vi "QueryTarget.vi"(8 "error in (no error)":errorcluster, 11 "Target Reference in":refnum<k24>) -> (0 "error out":errorcluster, 2 "Target Information":T1, 3 "Target Reference out":refnum<k24>)   [LabVIEW 2015, in "VeriStandTestUtilities.lvlib"]
uses:
  VeriStandTestUtilities.lvlib
  NationalInstruments.VeriStand.SystemDefinitionAPI
  TargetInformation.ctl
panel:
  in  "Target Information":T1
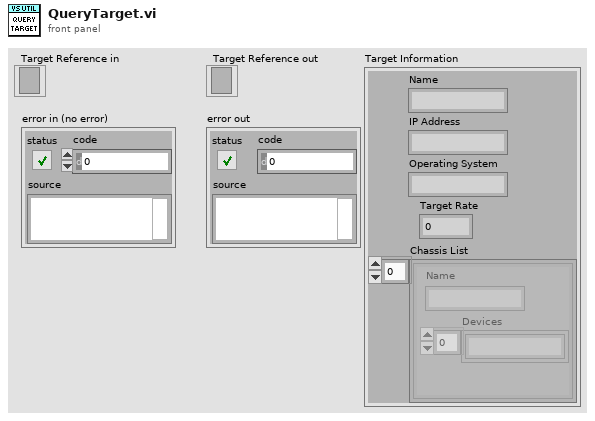
[diagram p1: front panel]
types:
  T1 = typedef "VeriStandTestUtilities.lvlib/TargetInformation.ctl" = cluster{"Name":string, "IP Address":string, "Operating System":string, "Target Rate":dbl, "Chassis List":cluster{"Name":string, "Devices":string[]}[]}
  T2 = typedef "VeriStandTestUtilities.lvlib/ChassisInformation.ctl" = cluster{"Name":string, "Devices":string[]}
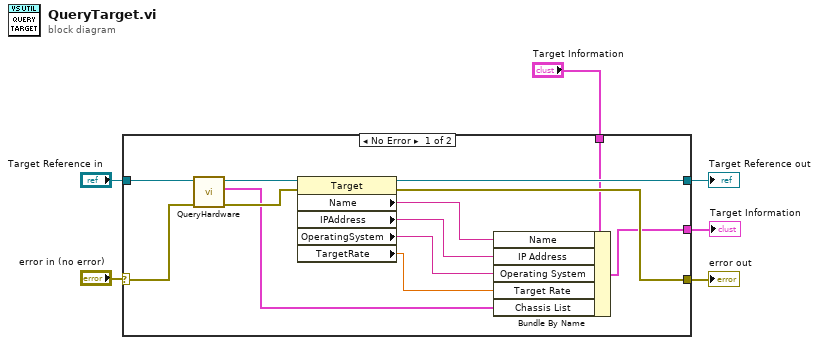
[diagram p0: block diagram]
diagram:
  n1 = case shown="No Error" "error in (no error)" {
    selector: "error in (no error)" -> [w18 w21]
    tunnel: [w19 w21] -> w5
    tunnel: "Target Reference in" -> [w10 w20]
    tunnel: [w17 w20] -> w3
    tunnel: "Target Information" -> [w16 _]
    tunnel: [w11 _] -> w1
    frame No Error {
      n2 = call "QueryHardware.vi"("error in (no error)"=w18, "Target Reference In"=w10) -> ("error out"=w8:errorcluster, "Chassis List out"=w7:T2[], "Target Reference out"=w9:refnum<k24>)  [unwired: 7 in]
      n3 = property class="Target"(reference=w9, error in=w8) -> (reference out=w17:refnum<k24>, error out=w19:errorcluster, "Name"=w15:string, "IPAddress"=w14:string, "OperatingSystem"=w13:string, "TargetRate"=w12:dbl)
      n4 = Bundle By Name(cluster=w16, "Name"=w15, "IP Address"=w14, "Operating System"=w13, "Target Rate"=w12, "Chassis List"=w7) -> (w11:T1)
    }
    frame Error {
    }
  }
  "error out" <- w5
  "Target Reference out" <- w3
  "Target Information" <- w1
